vi "Commit Transaction.vi"(8 "error in":errorcluster, 11 "DB-ADO in":refnum<class "DB-ADO.lvclass">) -> (0 "error out":errorcluster, 3 "DB-ADO out":refnum<class "DB-ADO.lvclass">)   [LabVIEW 2022 SP3, in "hse-db-ado.lvlib" / "DB-ADO.lvclass"]
doc: "Commit a transaction. Either all SQL-commands get commited or, in case of an error, all get rejected.\n\n____\nHAMPEL SOFTWARE ENGINEERING v1.4.0 (2023-12-19 09:52)"
uses:
  DB-ADO.lvclass
  DB-ADO.lvclass/DB-ADO.ctl
  ADO-DB-Drivers/ADO-DB-Driver.lvlib
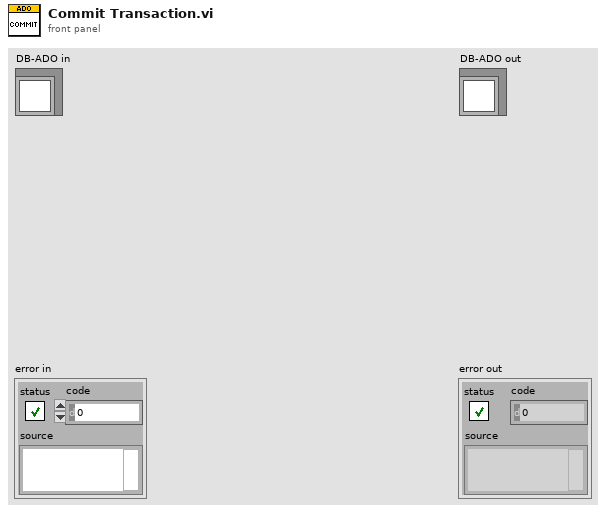
[diagram p1: front panel]
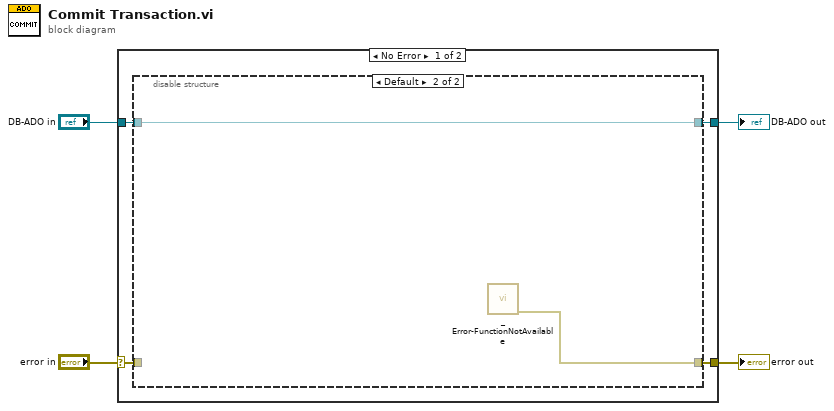
[diagram p0: block diagram]
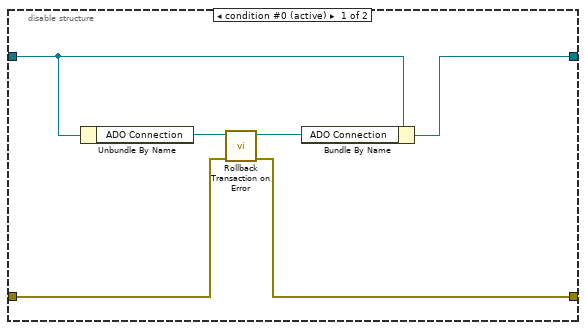
[diagram p2: hidden frame]
diagram:
  n1 = case shown="No Error" "error in" {
    selector: "error in" -> [w6 w18]
    tunnel: [w5 w18] -> w3
    tunnel: [w7 w17] -> w1
    tunnel: "DB-ADO in" -> [w8 w17]
    frame No Error {
      n2 = disable-structure shown="Default" {
        disable-tunnel: w8 -> [w13 w16]
        disable-tunnel: [w12 w16] -> w7
        disable-tunnel: w6 -> [w10 _]
        disable-tunnel: [w9 w15] -> w5
        frame condition #0 (active) {
          n3 = Unbundle By Name(w13) -> ("ADO Connection"=w14:refnum<k7>)
          n4 = call "Rollback Transaction on Error.vi"("error in"=w10, "Connection In"=w14) -> ("error out"=w9:errorcluster, "Connection Out"=w11:refnum<k7>)  [unwired: 7 in]
          n5 = Bundle By Name(cluster=w13, "ADO Connection"=w11) -> (w12:refnum<class "DB-ADO.lvclass">)
        }
        frame condition #1 {
          n6 = call "_Error-FunctionNotAvailable.vi"() -> ("error out"=w15:errorcluster)  [unwired: 11 in]
        }
      }
    }
    frame Error {
    }
  }
  "error out" <- w3
  "DB-ADO out" <- w1
